vi "FGV Pos.vi"(8 "error in (no error)":errorcluster, 10 "FGV Pos Data In":T1={"Portnumber"=0, "Position"=0.0, "Status"="", "Système ID"=1, "Connected axes"=[], "Velocity"=0.0, "Stage names"=[], "Device ID out"=0, "Servo"=FALSE} {"Système ID" min=1 max=10 step=1; "Portnumber" items=["COM1", "COM2", "COM3", "COM4", "COM5", "COM6", "COM7", "COM8", "COM9", "COM10", "COM11", "COM12", "COM13", "COM14", "COM15", "COM16", "COM17", "COM18", "COM19", "COM20", "COM21", "COM22", "COM23", "COM24", "COM25", "COM26", "COM27", "COM28", "COM29", "COM30"]}, 11 "Action":T2) -> (0 "error out":errorcluster, 3 "FGV Pos Data Out":T1={"Portnumber"=0, "Position"=0.0, "Status"="", "Système ID"=1, "Connected axes"=[], "Velocity"=0.0, "Stage names"=[], "Device ID out"=0, "Servo"=FALSE} {"Système ID" min=1 max=10 step=1; "Portnumber" items=["COM1", "COM2", "COM3", "COM4", "COM5", "COM6", "COM7", "COM8", "COM9", "COM10", "COM11", "COM12", "COM13", "COM14", "COM15", "COM16", "COM17", "COM18", "COM19", "COM20", "COM21", "COM22", "COM23", "COM24", "COM25", "COM26", "COM27", "COM28", "COM29", "COM30"]})   [LabVIEW 2013]
uses:
  Action Pos.ctl
  FGV Pos Data.ctl
  <userlib>/GCSLabView/Low Level/Communication.llb/Available interfaces.ctl
  <userlib>/GCSLabView/Low Level/Communication.llb/Available DLLs.ctl
  <userlib>/GCSLabView/Low Level/Communication.llb/Available DLL interfaces.ctl
  <userlib>/GCSLabView/Low Level/General command.llb/Controller names.ctl
  Slit/FGV/FGV Slit Data.ctl
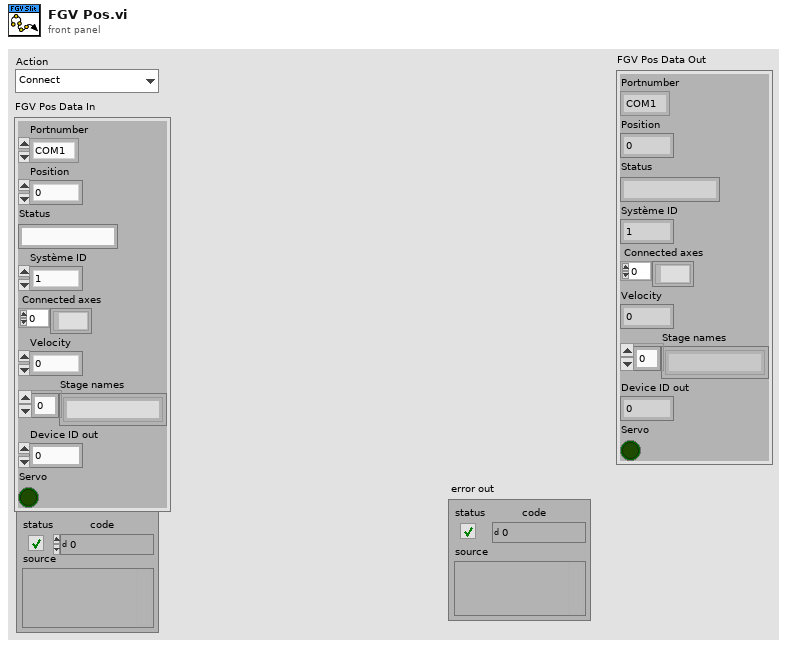
[diagram p1: front panel]
types:
  T1 = typedef "FGV Pos Data.ctl" = cluster{"Portnumber":i32, "Position":dbl, "Status":string, "Système ID":i32, "Connected axes":string[], "Velocity":dbl, "Stage names":string[], "Device ID out":i32, "Servo":bool}
  T2 = typedef "Action Pos.ctl" = enum16{"Connect", "Initialize", "Set Velocity", "Get Velocity", "Switch Servo", "Move Rel", "Move Abs", "Position", "Status", "Abort", "Disconnect"}
  T3 = typedef "FGV Slit Data.ctl" = cluster{"Portnumber":i32, "Position":dbl, "Status":string, "Système ID":i32, "Connected axes":string[], "Velocity":dbl, "Stage names":string[], "Device ID out":i32}
  T4 = typedef "Available interfaces.ctl" = u16
  T5 = cluster{"RS232 Portnumber":i32, "Timeout":i32, "RS232 Baud rate":u32, "Interface":T4, "GPIB Bus":i32, "GPIB Address":i32, "GPIB Mode":i32}
  T6 = cluster{"input XON/XOFF":bool, "input HW Handshake":bool, "input alt HW HShk":bool, "output XON/XOFF":bool, "output HW Handshake":bool, "output alt HW HShk":bool, "XOFF byte ":u8, "XON byte":u8, "parity error byte":u16}
  T7 = cluster{"data bits":u16, "stop bits":enum16{"1 bit", "1.5 bits", "2 bits"}, "parity":enum16{"no parity", "odd parity", "even parity", "mark parity", "space parity"}}
  T8 = typedef "Controller names.ctl" = enum16{"None", "Analog", "C-702", "C-843", "C-843.PM", "C-844", "C-848", "C-865", "C-866", "C-867", "C-880", "E-516", "E-517", "E-709", "E-710", "E-712", "E-725", "E-753", "E-755", "E-761", "E-816", "E-861", "F-206", "M-840", "M-850", "M-8X0", "Mercury", "Mercury_GCS"}
  T9 = typedef "Available DLLs.ctl" = u16
  T10 = typedef "Available DLL interfaces.ctl" = u16
  T11 = cluster{"DLL for Device":T9, "DLL Interface":T10, "Parameter":string}
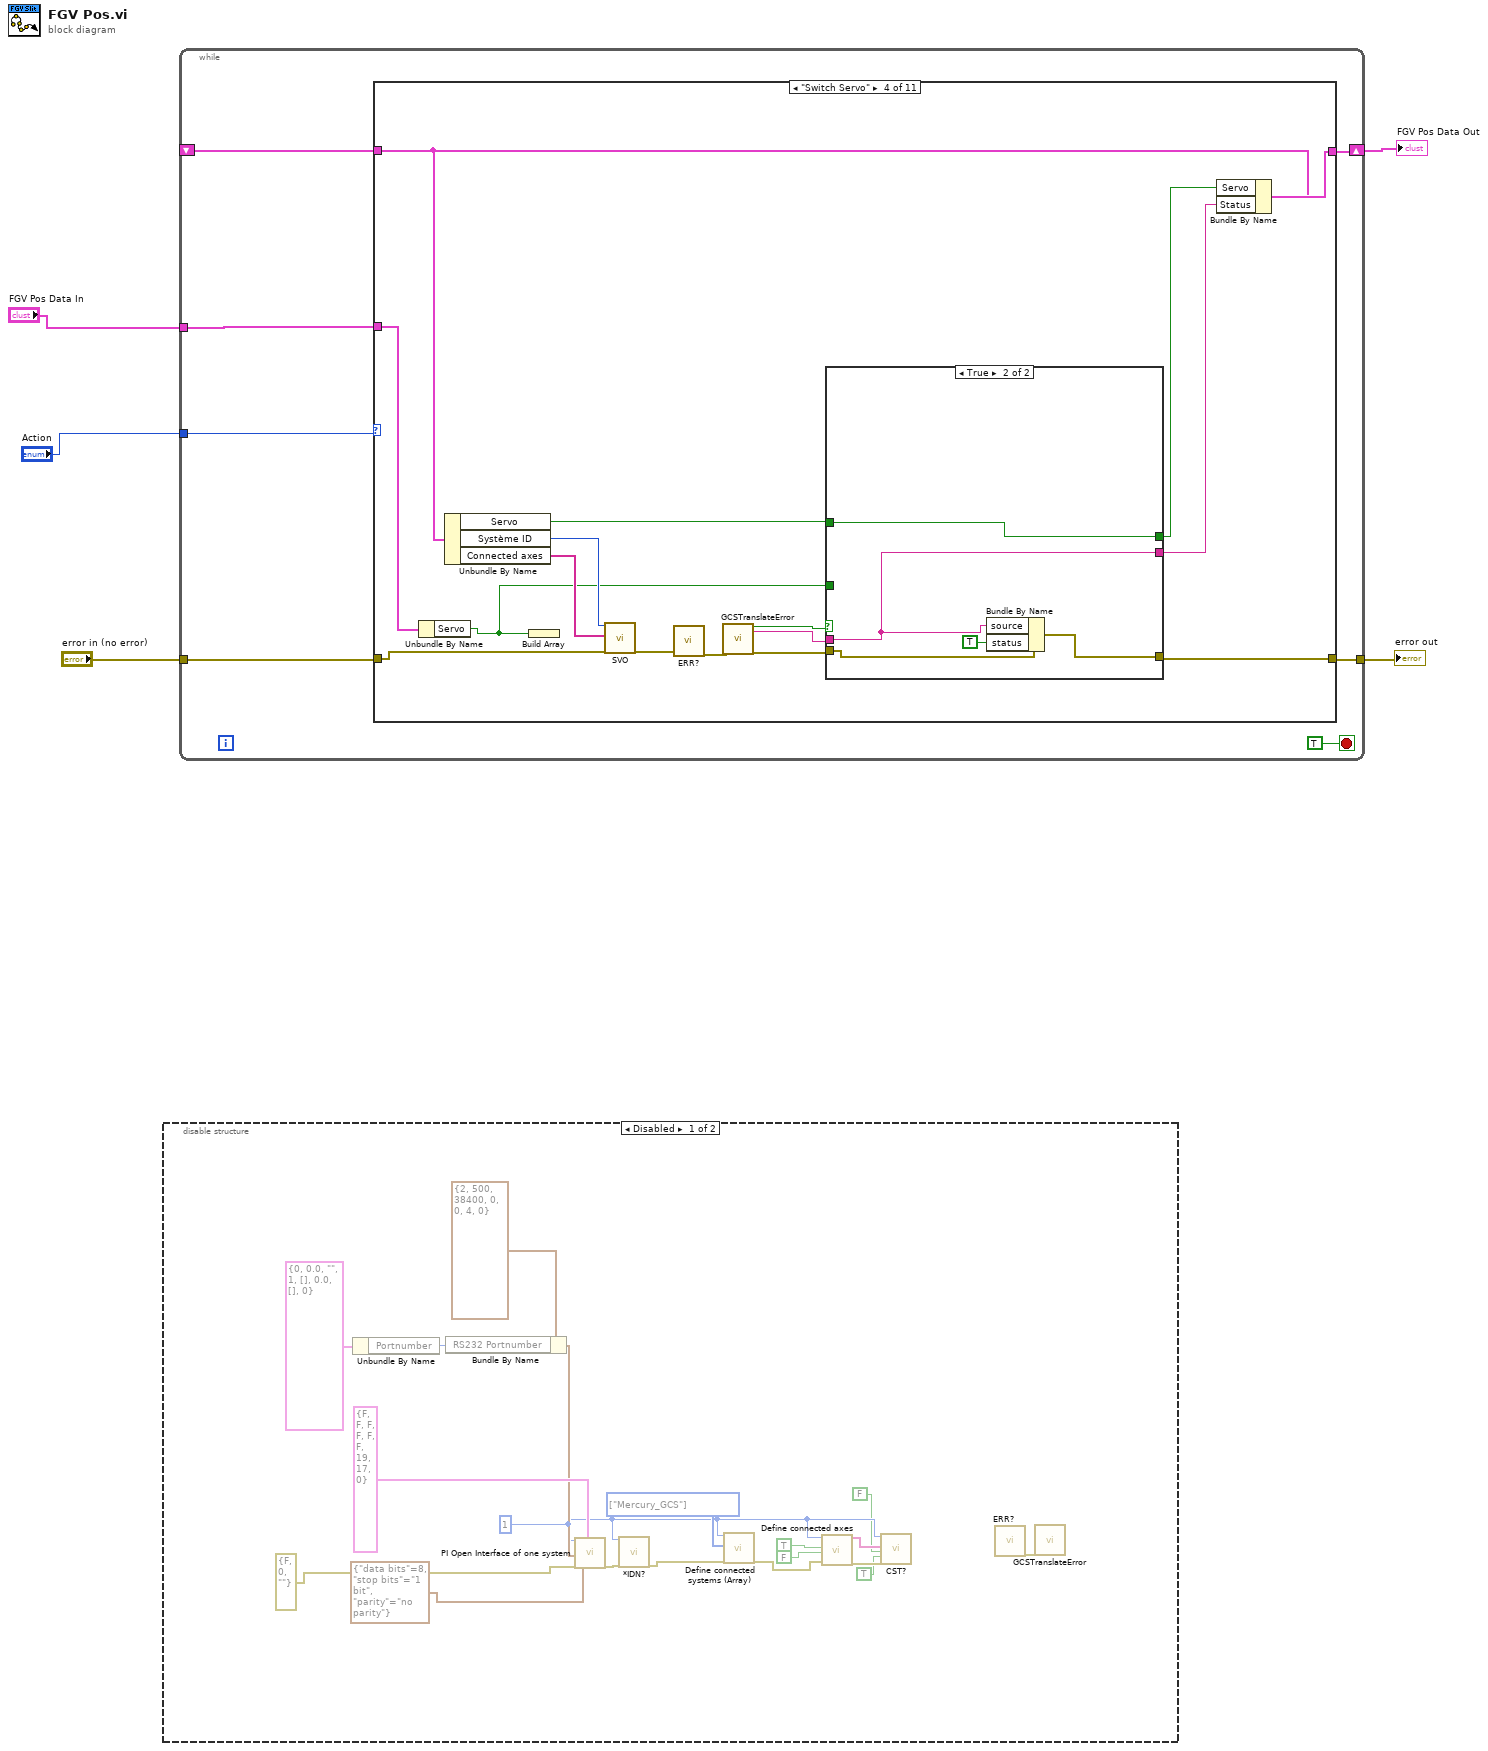
[diagram p0: block diagram]
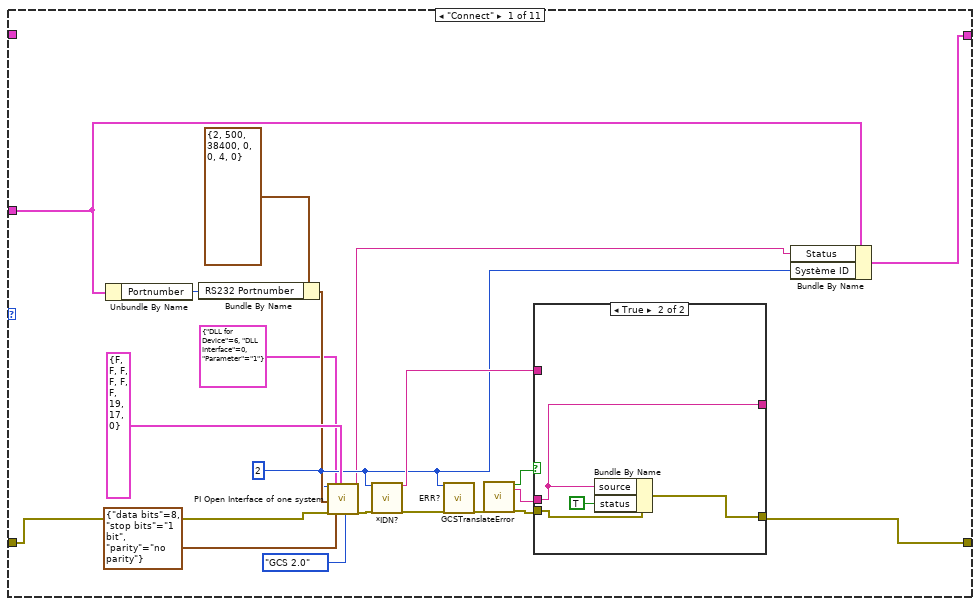
[diagram p3: hidden frame]
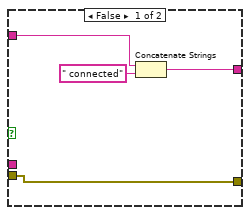
[diagram p4: hidden frame]
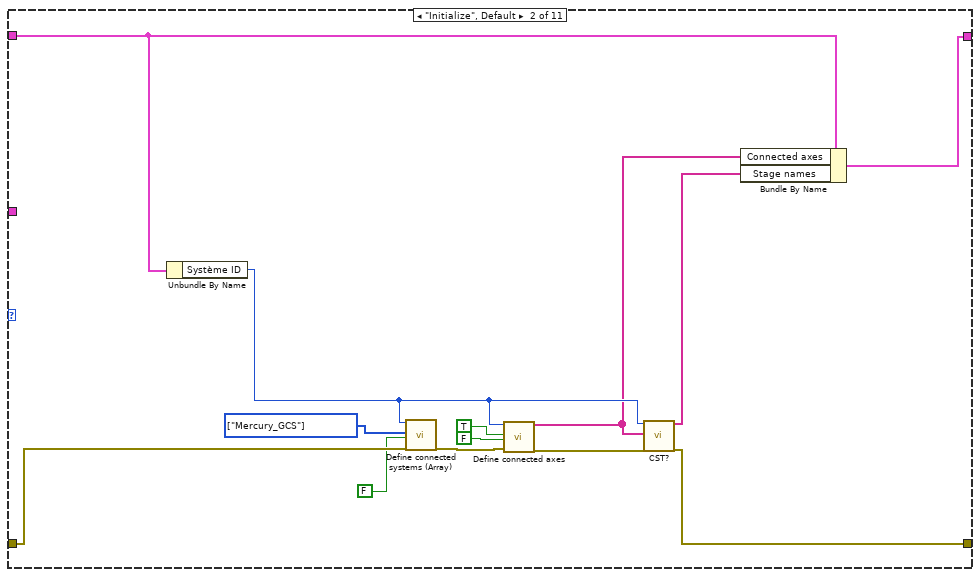
[diagram p5: hidden frame]
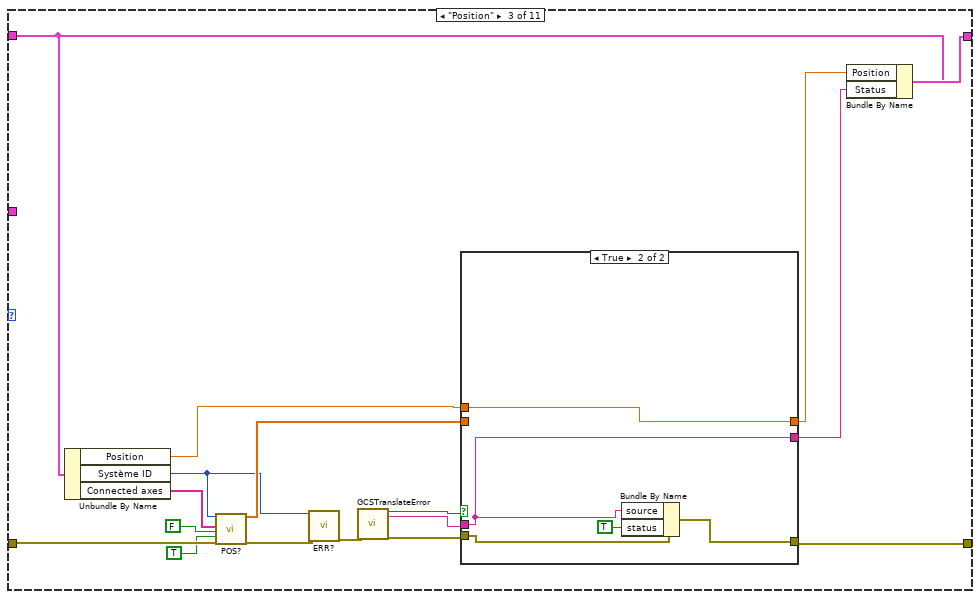
[diagram p6: hidden frame]
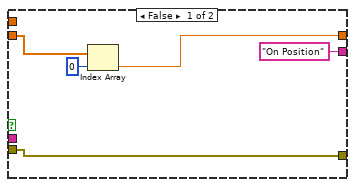
[diagram p7: hidden frame]
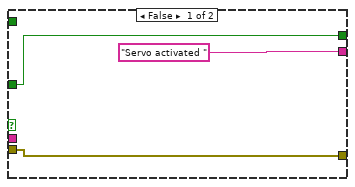
[diagram p8: hidden frame]
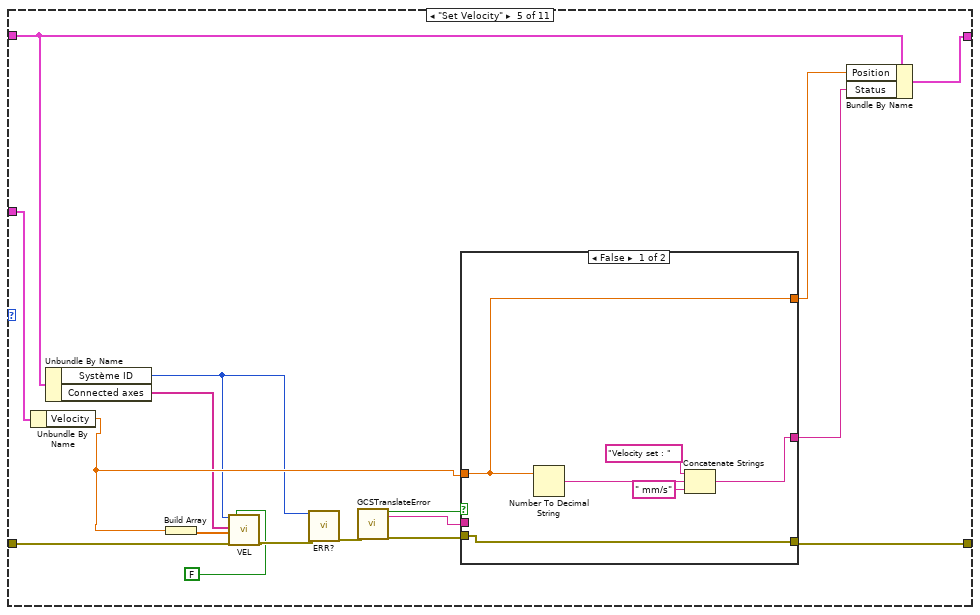
[diagram p9: hidden frame]
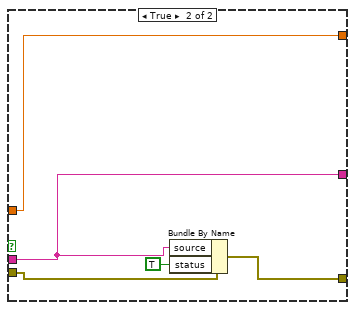
[diagram p10: hidden frame]
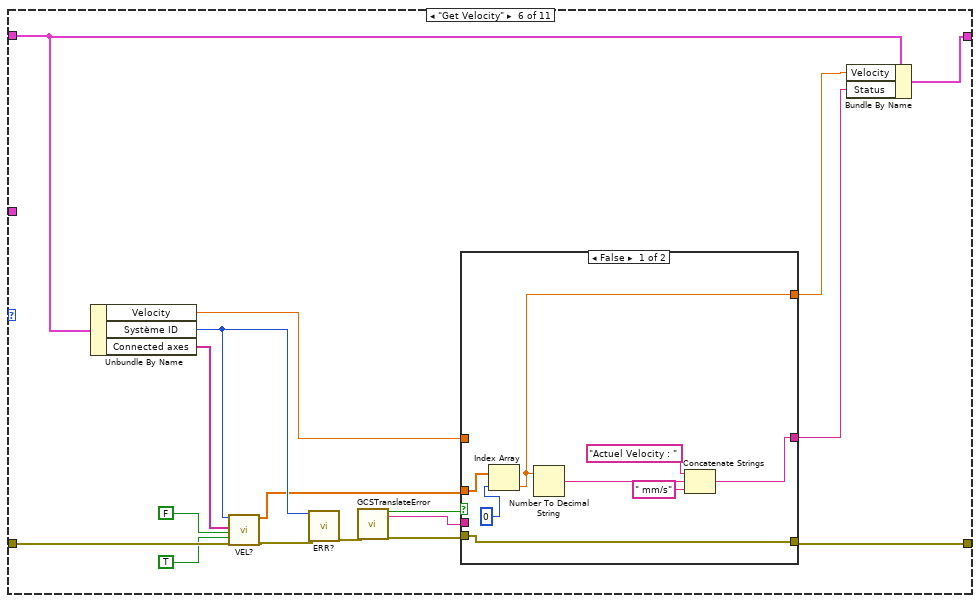
[diagram p11: hidden frame]
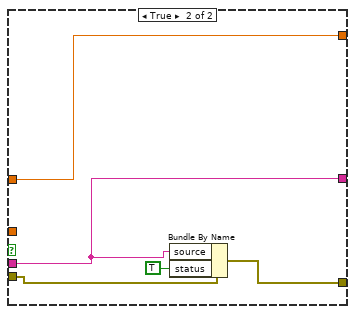
[diagram p12: hidden frame]
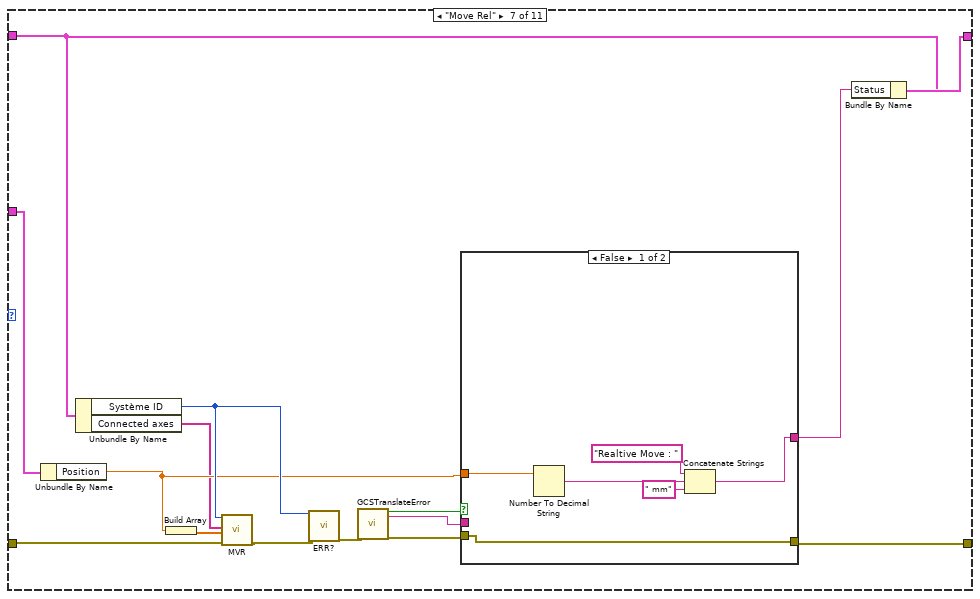
[diagram p13: hidden frame]
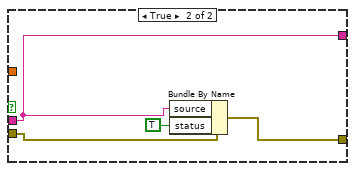
[diagram p14: hidden frame]
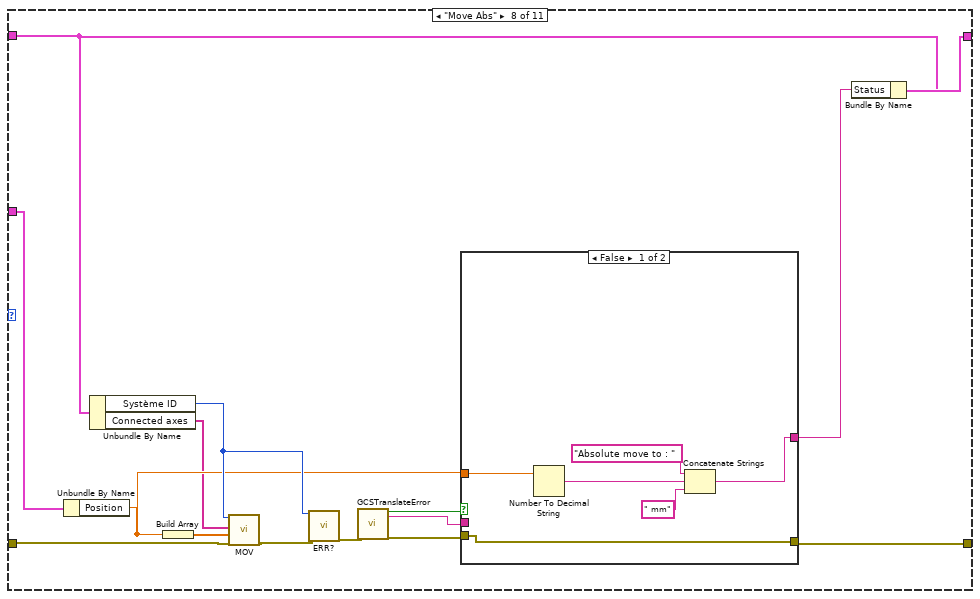
[diagram p15: hidden frame]
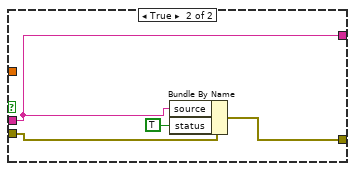
[diagram p16: hidden frame]
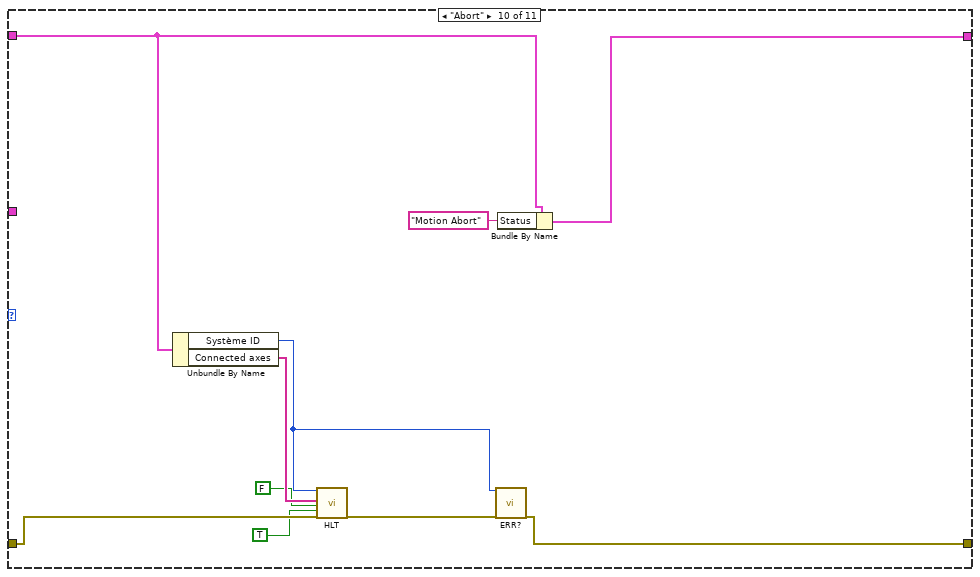
[diagram p18: hidden frame]
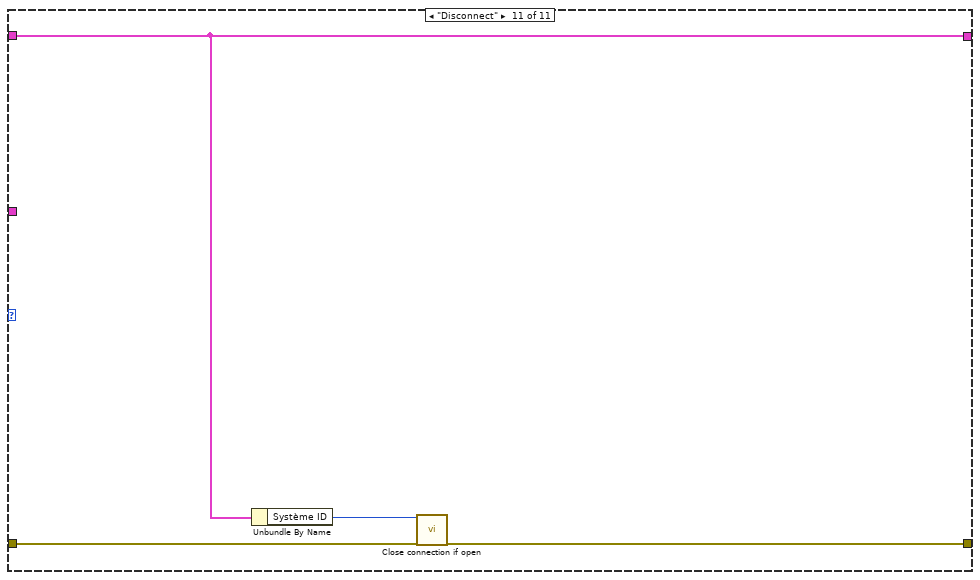
[diagram p19: hidden frame]
diagram:
  n1 = disable-structure shown="Disabled" {
    frame Disabled {
      w18 = T8[] [enum."Mercury_GCS"] items=["None", "Analog", "C-702", "C-843", "C-843.PM", "C-844", "C-848", "C-865", "C-866", "C-867", "C-880", "E-516", "E-517", "E-709", "E-710", "E-712", "E-725", "E-753", "E-755", "E-761", "E-816", "E-861", "F-206", "M-840", "M-850", "M-8X0", "Mercury", "Mercury_GCS"] ("Controller names")
      w10 = 1 ("System number")
      n2 = Unbundle By Name(T3 {"Portnumber"=0, "Position"=0.0, "Status"="", "Système ID"=1, "Connected axes"=[], "Velocity"=0.0, "Stage names"=[], "Device ID out"=0} ("input cluster")) -> ("Portnumber"=w20:i32)
      n3 = Bundle By Name(cluster=T5 {"RS232 Portnumber"=2, "Timeout"=500, "RS232 Baud rate"=38400, "Interface"=0, "GPIB Bus"=0, "GPIB Address"=4, "GPIB Mode"=0} ("Interface configuration"), "RS232 Portnumber"=w20) -> (w19:T5)
      n4 = call <userlib>:"PI Open Interface of one system.vi"("System number"=w10, "Interface configuration"=w19, "error in"=errorcluster {"status"=FALSE, "code"=0, "source"=""}, "Bit settings and parity"=T7 {"data bits"=8, "stop bits"=enum."1 bit", "parity"=enum."no parity"}, "Flow control"=T6 {"input XON/XOFF"=FALSE, "input HW Handshake"=FALSE, "input alt HW HShk"=FALSE, "output XON/XOFF"=FALSE, "output HW Handshake"=FALSE, "output alt HW HShk"=FALSE, "XOFF byte "=19, "XON byte"=17, "parity error byte"=0}) -> ("error out"=w22:errorcluster)  [unwired: 13 in, 1 out]
      n5 = call <userlib>:"*IDN?.vi"("System no."=w10, "error in"=w22) -> ("error out"=w14:errorcluster)  [unwired: 16 in, 1 out]
      n6 = call <userlib>:"Define connected systems (Array).vi"("System no."=w10, "Controller names"=w18, "error in"=w14) -> ("error out"=w11:errorcluster)  [unwired: 16 in]
      n7 = call <userlib>:"Define connected axes.vi"("System no."=w10, "Read from\ncontroller?"=TRUE ("Read from\ncontroller?"), "Invert\norder?"=FALSE ("Invert\norder?"), "error in"=w11) -> ("Conn. Axes out"=w9:string[], "error out"=w8:errorcluster)  [unwired: 14 in]
      n8 = call <userlib>:"CST?.vi"("System no."=w10, "Axes to query"=w9, "All Axes?"=FALSE, "Axis Identifier?"=TRUE, "error in"=w8) -> ()  [unwired: 13 in, 2 out]
      n9 = call <userlib>:"ERR?.vi"() -> ("error out"=w24:errorcluster)  [unwired: 18 in, 1 out]
      n10 = call <userlib>:"GCSTranslateError.vi"("error in"=w24) -> ()  [unwired: 16 in, 3 out]
    }
    frame Enabled {
    }
  }
  n11 = while {
    tunnel: "Action" -> [w30]
    tunnel: "FGV Pos Data In" -> [w29]
    shift-right: [w28] -> w1
    shift-left: _ -> [w25]
    tunnel: "error in (no error)" -> [w27]
    tunnel: [w26] -> w4
    stop <- TRUE stop-if-true
    n12 = case shown="\"Switch Servo\"" w30 {
      tunnel: w29 -> [w48 _ _ w102 w129 _ w184 w209 _ _ _]
      tunnel: [w50 w62 w85 w111 w136 w164 w192 w217 w233 w237 w246] -> w28
      tunnel: w25 -> [_ w64 w81 w109 w126 w154 w185 w210 w233 w239 w246]
      tunnel: w27 -> [w49 w67 w83 w106 w132 w160 w189 w213 w232 w243 w247]
      tunnel: [w51 w66 w84 w110 w135 w163 w191 w216 w232 w241 w244] -> w26
      frame "Connect" {
        w36 = 2 ("System number")
        n13 = Unbundle By Name(w48) -> ("Portnumber"=w38:i32)
        n14 = Bundle By Name(cluster=T5 {"RS232 Portnumber"=2, "Timeout"=500, "RS232 Baud rate"=38400, "Interface"=0, "GPIB Bus"=0, "GPIB Address"=4, "GPIB Mode"=0} ("Interface configuration"), "RS232 Portnumber"=w38) -> (w37:T5)
        n15 = call <userlib>:"PI Open Interface of one system.vi"("System number"=w36, "Interface configuration"=w37, "error in"=w49, "DLL Interface\nConfiguration"=T11 {"DLL for Device"=6, "DLL Interface"=0, "Parameter"="1"} ("DLL Interface\nConfiguration"), "Bit settings and parity"=T7 {"data bits"=8, "stop bits"=enum."1 bit", "parity"=enum."no parity"}, "Flow control"=T6 {"input XON/XOFF"=FALSE, "input HW Handshake"=FALSE, "input alt HW HShk"=FALSE, "output XON/XOFF"=FALSE, "output HW Handshake"=FALSE, "output alt HW HShk"=FALSE, "XOFF byte "=19, "XON byte"=17, "parity error byte"=0}, "Syntax"=enum16{"GCS 1.0", "GCS 2.0"}."GCS 2.0") -> ("String read"=w33:string, "error out"=w41:errorcluster)  [unwired: 11 in]
        n16 = call <userlib>:"*IDN?.vi"("System no."=w36, "error in"=w41) -> ("Identification"=w40:string, "error out"=w35:errorcluster)  [unwired: 16 in]
        n17 = call <userlib>:"ERR?.vi"("System no."=w36, "error in"=w35) -> ("error out"=w47:errorcluster)  [unwired: 16 in, 1 out]
        n18 = call <userlib>:"GCSTranslateError.vi"("error in"=w47) -> ("GCS Error?"=w46:bool, "Error Description"=w45:string, "error out"=w44:errorcluster)  [unwired: 16 in]
        n19 = case shown="True" w46 {
          tunnel: w40 -> [w55 _]
          tunnel: [w52 w58] -> w51
          tunnel: [w53 w57] -> _
          tunnel: w45 -> [_ w57]
          tunnel: w44 -> [w52 w59]
          frame False {
            n20 = Concatenate Strings(w55, " connected" ("string")) -> (w53:string)
          }
          frame True {
            n21 = Bundle By Name(cluster=w59, "source"=w57, "status"=TRUE) -> (w58:errorcluster)
          }
        }
        n22 = Bundle By Name(cluster=w48, "Status"=w33, "Système ID"=w36) -> (w50:T1)
      }
      frame "Initialize", Default {
        w72 = T8[] [enum."Mercury_GCS"] items=["None", "Analog", "C-702", "C-843", "C-843.PM", "C-844", "C-848", "C-865", "C-866", "C-867", "C-880", "E-516", "E-517", "E-709", "E-710", "E-712", "E-725", "E-753", "E-755", "E-761", "E-816", "E-861", "F-206", "M-840", "M-850", "M-8X0", "Mercury", "Mercury_GCS"] ("Controller names")
        n23 = Unbundle By Name(w64) -> ("Système ID"=w65:i32)
        n24 = call <userlib>:"Define connected systems (Array).vi"("System no."=w65, "Controller names"=w72, "Change only one system?"=FALSE, "error in"=w67) -> ("error out"=w69:errorcluster)  [unwired: 15 in]
        n25 = call <userlib>:"Define connected axes.vi"("System no."=w65, "Read from\ncontroller?"=TRUE ("Read from\ncontroller?"), "Invert\norder?"=FALSE ("Invert\norder?"), "error in"=w69) -> ("Conn. Axes out"=w60:string[], "error out"=w68:errorcluster)  [unwired: 14 in]
        n26 = call <userlib>:"CST?.vi"("System no."=w65, "Axes to query"=w60, "error in"=w68) -> ("Stage names"=w63:string[], "error out"=w66:errorcluster)  [unwired: 15 in]
        n27 = Bundle By Name(cluster=w64, "Connected axes"=w60, "Stage names"=w63) -> (w62:T1)
      }
      frame "Position" {
        n28 = Unbundle By Name(w81) -> ("Position"=w79:dbl, "Système ID"=w75:i32, "Connected axes"=w76:string[])
        n29 = call <userlib>:"POS?.vi"("System no."=w75, "Axes to query"=w76, "All axes?"=FALSE, "Axis identifier?"=TRUE, "error in"=w83) -> ("Position"=w80:dbl[], "error out"=w82:errorcluster)  [unwired: 13 in]
        n30 = call <userlib>:"ERR?.vi"("System no."=w75, "error in"=w82) -> ("error out"=w89:errorcluster)  [unwired: 16 in, 1 out]
        n31 = call <userlib>:"GCSTranslateError.vi"("error in"=w89) -> ("GCS Error?"=w88:bool, "Error Description"=w87:string, "error out"=w86:errorcluster)  [unwired: 16 in]
        n32 = case shown="True" w88 {
          tunnel: [w94 w98] -> w84
          tunnel: ["On Position" ("Error Description") w97] -> w78
          tunnel: w87 -> [_ w97]
          tunnel: w86 -> [w94 w99]
          tunnel: w80 -> [w92 _]
          tunnel: [w90 w95] -> w77
          tunnel: w79 -> [_ w95]
          frame False {
            n33 = Index Array(array=w92, index=0) -> (element=w90:dbl)
          }
          frame True {
            n34 = Bundle By Name(cluster=w99, "source"=w97, "status"=TRUE) -> (w98:errorcluster)
          }
        }
        n35 = Bundle By Name(cluster=w81, "Position"=w77, "Status"=w78) -> (w85:T1)
      }
      frame "Switch Servo" {
        n36 = Unbundle By Name(w102) -> ("Servo"=w101:bool)
        n37 = Unbundle By Name(w109) -> ("Servo"=w100:bool, "Système ID"=w104:i32, "Connected axes"=w103:string[])
        n38 = Build Array(w101) -> ()  [unwired: 1 out]
        n39 = call <userlib>:"SVO.vi"("System no."=w104, "Axes to command"=w103, "error in"=w106) -> ("error out"=w105:errorcluster)  [unwired: 16 in]
        n40 = call <userlib>:"ERR?.vi"("error in"=w105) -> ("error out"=w115:errorcluster)  [unwired: 17 in, 1 out]
        n41 = call <userlib>:"GCSTranslateError.vi"("error in"=w115) -> ("GCS Error?"=w114:bool, "Error Description"=w113:string, "error out"=w112:errorcluster)  [unwired: 16 in]
        n42 = case shown="True" w114 {
          tunnel: [w118 w122] -> w110
          tunnel: ["Servo activated " ("Error Description") w121] -> w108
          tunnel: w113 -> [_ w121]
          tunnel: w112 -> [w118 w123]
          tunnel: [w116 w119] -> w107
          tunnel: w100 -> [_ w119]
          tunnel: w101 -> [w116 _]
          frame False {
          }
          frame True {
            n43 = Bundle By Name(cluster=w123, "source"=w121, "status"=TRUE) -> (w122:errorcluster)
          }
        }
        n44 = Bundle By Name(cluster=w109, "Servo"=w107, "Status"=w108) -> (w111:T1)
      }
      frame "Set Velocity" {
        n45 = Unbundle By Name(w129) -> ("Velocity"=w128:dbl)
        n46 = Unbundle By Name(w126) -> ("Système ID"=w127:i32, "Connected axes"=w124:string[])
        n47 = Build Array(w128) -> (w133:dbl[])
        n48 = call <userlib>:"VEL.vi"("System no."=w127, "Axes to set"=w124, "Velocity values"=w133, "error in"=w132, "Without axis ID?"=FALSE) -> ("error out"=w131:errorcluster)  [unwired: 13 in, 1 out]
        n49 = call <userlib>:"ERR?.vi"("System no."=w127, "error in"=w131) -> ("error out"=w140:errorcluster)  [unwired: 16 in, 1 out]
        n50 = call <userlib>:"GCSTranslateError.vi"("error in"=w140) -> ("GCS Error?"=w139:bool, "Error Description"=w138:string, "error out"=w137:errorcluster)  [unwired: 16 in]
        n51 = case shown="False" w139 {
          tunnel: [w146 w150] -> w135
          tunnel: [w143 w149] -> w134
          tunnel: w138 -> [_ w149]
          tunnel: w137 -> [w146 w151]
          tunnel: w128 -> [w141 w147]
          tunnel: [w141 w147] -> w130
          frame False {
            n52 = Number To Decimal String(number=w141) -> (decimal integer string=w145:string)  [unwired: 1 in]
            n53 = Concatenate Strings("Velocity set : " ("Error Description"), w145, " mm/s" ("string")) -> (w143:string)
          }
          frame True {
            n54 = Bundle By Name(cluster=w151, "source"=w149, "status"=TRUE) -> (w150:errorcluster)
          }
        }
        n55 = Bundle By Name(cluster=w126, "Position"=w130, "Status"=w134) -> (w136:T1)
      }
      frame "Get Velocity" {
        n56 = Unbundle By Name(w154) -> ("Velocity"=w155:dbl, "Système ID"=w161:i32, "Connected axes"=w157:string[])
        n57 = call <userlib>:"VEL?.vi"("System no."=w161, "Axes to query"=w157, "All axes?"=FALSE, "Axis identifier?"=TRUE, "error in"=w160) -> ("Velocity"=w158:dbl[], "error out"=w159:errorcluster)  [unwired: 13 in]
        n58 = call <userlib>:"ERR?.vi"("System no."=w161, "error in"=w159) -> ("error out"=w168:errorcluster)  [unwired: 16 in, 1 out]
        n59 = call <userlib>:"GCSTranslateError.vi"("error in"=w168) -> ("GCS Error?"=w167:bool, "Error Description"=w166:string, "error out"=w165:errorcluster)  [unwired: 16 in]
        n60 = case shown="False" w167 {
          tunnel: [w176 w180] -> w163
          tunnel: [w173 w179] -> w162
          tunnel: w166 -> [_ w179]
          tunnel: w165 -> [w176 w181]
          tunnel: w158 -> [w171 _]
          tunnel: [w169 w177] -> w156
          tunnel: w155 -> [_ w177]
          frame False {
            n61 = Index Array(array=w171, index=i16 0 ("width (-)")) -> (element=w169:dbl)
            n62 = Number To Decimal String(number=w169) -> (decimal integer string=w175:string)  [unwired: 1 in]
            n63 = Concatenate Strings("Actuel Velocity : " ("Error Description"), w175, " mm/s" ("string")) -> (w173:string)
          }
          frame True {
            n64 = Bundle By Name(cluster=w181, "source"=w179, "status"=TRUE) -> (w180:errorcluster)
          }
        }
        n65 = Bundle By Name(cluster=w154, "Velocity"=w156, "Status"=w162) -> (w164:T1)
      }
      frame "Move Rel" {
        n66 = Unbundle By Name(w184) -> ("Position"=w183:dbl)
        n67 = Unbundle By Name(w185) -> ("Système ID"=w186:i32, "Connected axes"=w182:string[])
        n68 = Build Array(w183) -> (w187:dbl[])
        n69 = call <userlib>:"MVR.vi"("System no."=w186, "Axes to move"=w182, "Position values"=w187, "error in"=w189) -> ("error out"=w188:errorcluster)  [unwired: 15 in]
        n70 = call <userlib>:"ERR?.vi"("System no."=w186, "error in"=w188) -> ("error out"=w196:errorcluster)  [unwired: 16 in, 1 out]
        n71 = call <userlib>:"GCSTranslateError.vi"("error in"=w196) -> ("GCS Error?"=w195:bool, "Error Description"=w194:string, "error out"=w193:errorcluster)  [unwired: 16 in]
        n72 = case shown="False" w195 {
          tunnel: [w202 w205] -> w191
          tunnel: [w198 w204] -> w190
          tunnel: w194 -> [_ w204]
          tunnel: w193 -> [w202 w206]
          tunnel: w183 -> [w201 _]
          frame False {
            n73 = Number To Decimal String(number=w201) -> (decimal integer string=w200:string)  [unwired: 1 in]
            n74 = Concatenate Strings("Realtive Move : " ("Error Description"), w200, " mm" ("string")) -> (w198:string)
          }
          frame True {
            n75 = Bundle By Name(cluster=w206, "source"=w204, "status"=TRUE) -> (w205:errorcluster)
          }
        }
        n76 = Bundle By Name(cluster=w185, "Status"=w190) -> (w192:T1)
      }
      frame "Move Abs" {
        n77 = Unbundle By Name(w209) -> ("Position"=w208:dbl)
        n78 = Unbundle By Name(w210) -> ("Système ID"=w211:i32, "Connected axes"=w207:string[])
        n79 = Build Array(w208) -> (w212:dbl[])
        n80 = call <userlib>:"MOV.vi"("System no."=w211, "Axes to move"=w207, "Position values"=w212, "error in"=w213) -> ("error out"=w214:errorcluster)  [unwired: 15 in]
        n81 = call <userlib>:"ERR?.vi"("System no."=w211, "error in"=w214) -> ("error out"=w221:errorcluster)  [unwired: 16 in, 1 out]
        n82 = call <userlib>:"GCSTranslateError.vi"("error in"=w221) -> ("GCS Error?"=w220:bool, "Error Description"=w219:string, "error out"=w218:errorcluster)  [unwired: 16 in]
        n83 = case shown="False" w220 {
          tunnel: [w227 w230] -> w216
          tunnel: [w223 w229] -> w215
          tunnel: w219 -> [_ w229]
          tunnel: w218 -> [w227 w231]
          tunnel: w208 -> [w226 _]
          frame False {
            n84 = Number To Decimal String(number=w226) -> (decimal integer string=w225:string)  [unwired: 1 in]
            n85 = Concatenate Strings("Absolute move to : " ("Error Description"), w225, " mm" ("string")) -> (w223:string)
          }
          frame True {
            n86 = Bundle By Name(cluster=w231, "source"=w229, "status"=TRUE) -> (w230:errorcluster)
          }
        }
        n87 = Bundle By Name(cluster=w210, "Status"=w215) -> (w217:T1)
      }
      frame "Status" {
      }
      frame "Abort" {
        n88 = Unbundle By Name(w239) -> ("Système ID"=w240:i32, "Connected axes"=w236:string[])
        n89 = call <userlib>:"HLT.vi"("System no."=w240, "Affected axes"=w236, "All axes?"=FALSE, "Axis identifier?"=TRUE, "error in"=w243) -> ("error out"=w242:errorcluster)  [unwired: 14 in]
        n90 = call <userlib>:"ERR?.vi"("System no."=w240, "error in"=w242) -> ("error out"=w241:errorcluster)  [unwired: 16 in, 1 out]
        n91 = Bundle By Name(cluster=w239, "Status"="Motion Abort") -> (w237:T1)
      }
      frame "Disconnect" {
        n92 = Unbundle By Name(w246) -> ("Système ID"=w245:i32)
        n93 = call <userlib>:"Close connection if open.vi"("System no."=w245, "error in"=w247) -> ("error out"=w244:errorcluster)  [unwired: 16 in, 1 out]
      }
    }
  }
  "error out" <- w4
  "FGV Pos Data Out" <- w1
